vi "Control Auton Selection.vi"(11 "Driver Buttons":T1) -> (3 "Selection controls":cluster{"Up":bool, "Down":bool})   [LabVIEW 2013]
uses:
  <vilib>/Rock Robotics/WPI/Joystick/WPI_JoystickButtonState.ctl
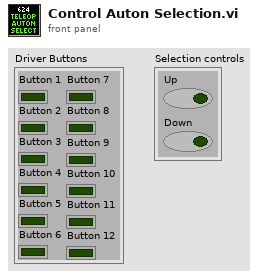
[diagram p1: front panel]
types:
  T1 = typedef "WPI_JoystickButtonState.ctl" = cluster{"Button 1":bool, "Button 2":bool, "Button 3":bool, "Button 4":bool, "Button 5":bool, "Button 6":bool, "Button 7":bool, "Button 8":bool, "Button 9":bool, "Button 10":bool, "Button 11":bool, "Button 12":bool}
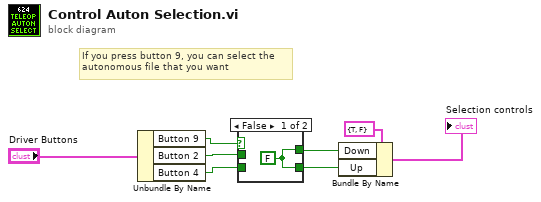
[diagram p0: block diagram]
diagram:
  # "If you press button 9, you can select the\nautonomous file that you want"
  n1 = Unbundle By Name("Driver Buttons") -> ("Button 9"=w2:bool, "Button 2"=w6:bool, "Button 4"=w5:bool)
  n2 = case shown="False" w2 {
    tunnel: [w9 w11] -> w7
    tunnel: w5 -> [_ w11]
    tunnel: [w9 w10] -> w8
    tunnel: w6 -> [_ w10]
    frame False {
      w9 = FALSE
    }
    frame True {
    }
  }
  n3 = Bundle By Name(cluster=cluster{"Up":bool, "Down":bool} {"Up"=TRUE, "Down"=FALSE} ("Selection controls"), "Down"=w8, "Up"=w7) -> (→"Selection controls":cluster{"Up":bool, "Down":bool})
